vi "Parse-attribute.vi"(8 "error in (no error)":errorcluster, 10 "String in":string, 11 "LaserPower in":refnum<class "LaserPower.lvclass">) -> (0 "error out":errorcluster, 1 "Valid attribute?":bool, 2 "Remaining string":string, 3 "LaserPower out":refnum<class "LaserPower.lvclass">)   [LabVIEW 2013, in "MaterialCharacterization.lvlib" / "LaserPower.lvclass"]
uses:
  LaserPower.lvclass
  Attributes.ctl
  Attribute-ID.ctl
  Attribute-XML.lvclass/Attribute-XML.ctl
  ID.lvclass/ID.ctl
  LaserPower.lvclass/LaserPower.ctl
  Write Attribute.vi
  Write ID-attribute.vi
  Write Power.vi
  Attribute-XML.lvclass
  ID.lvclass
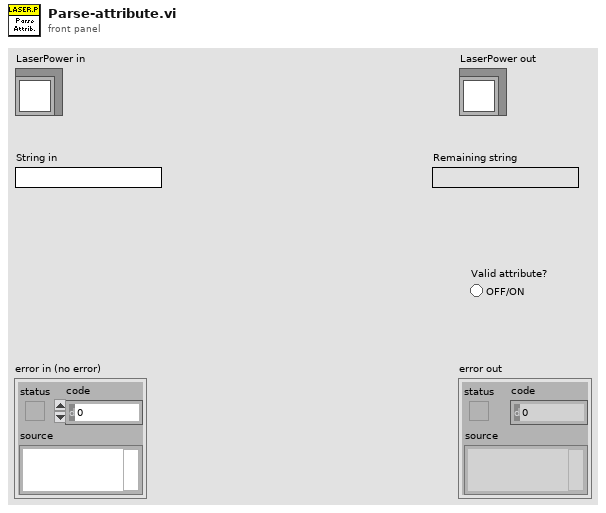
[diagram p1: front panel]
types:
  T1 = typedef "MaterialCharacterization.lvlib/ID.lvclass/Attribute-ID.ctl" = enum16{"FieldOffset", "TransformEnable", "Transform", "Units", "XYCalFactor", "EnableLaser", "JumpDelay", "MarkDelay", "PolyDelay", "LaserOnDelay", "LaserOffDelay", "JumpSpeed", "MarkSpeed", "LaserPowerDelay", "LaserEnableDelay", "LaserPower", "Offset"}
  T2 = typedef "MaterialCharacterization.lvlib/Attribute-XML.lvclass/Attributes.ctl" = enum16{"id"}
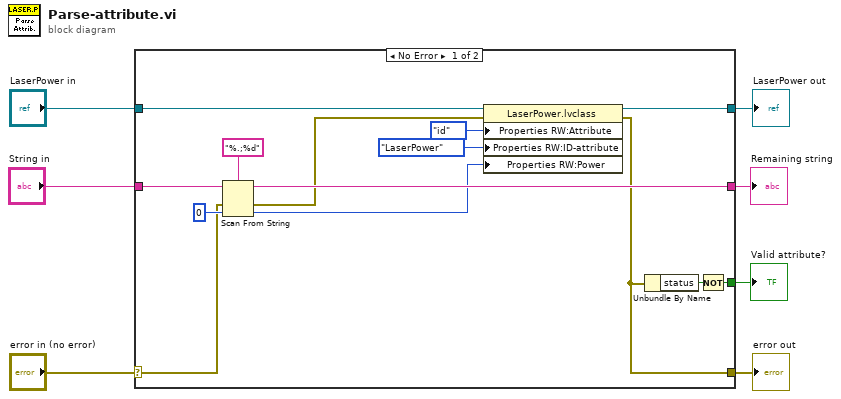
[diagram p0: block diagram]
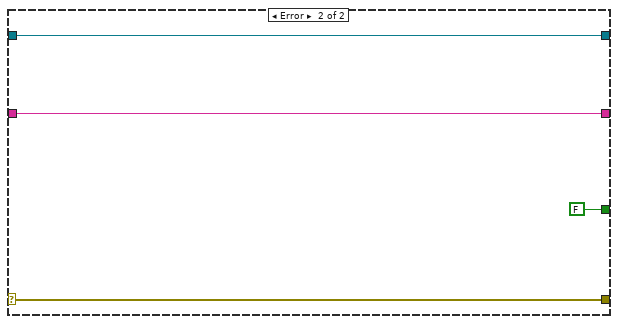
[diagram p2: hidden frame]
diagram:
  n1 = case shown="No Error" "error in (no error)" {
    selector: "error in (no error)" -> [w15 w25]
    tunnel: [w13 w25] -> w6
    tunnel: [w14 w24] -> w4
    tunnel: "LaserPower in" -> [w12 w24]
    tunnel: "String in" -> [w19 w23]
    tunnel: [w17 w23] -> w2
    tunnel: [w16 FALSE] -> w1
    frame No Error {
      n2 = Scan From String(format string="%.;%d", input string=w19, error in=w15, default 1=i64 0 ("default value 2")) -> (remaining string=w17:string, error out=w8:errorcluster, output 1=w11:i64)  [unwired: 1 in, 1 out]
      n3 = property class="LaserPower.lvclass"(reference=w12, error in=w8, "Properties RW:Attribute"=Attributes."id" ("Attribute"), "Properties RW:ID-attribute"=Attribute-ID."LaserPower" ("ID-attribute"), "Properties RW:Power"=w11) -> (reference out=w14:refnum<class "LaserPower.lvclass">, error out=w13:errorcluster)
      n4 = Unbundle By Name(w13) -> ("status"=w20:bool)
      n5 = Not(x=w20) -> (.not. x?=w16:bool)
    }
    frame Error {
    }
  }
  "error out" <- w6
  "LaserPower out" <- w4
  "Remaining string" <- w2
  "Valid attribute?" <- w1
